vi "Build Waveform Settings.vi"(8 "error in":errorcluster, 11 "Node Ptr":T1 format="%.0x") -> (0 "error out":errorcluster, 2 "Waveform Settings Table":string[][](array[string]), 3 "Node Ptr out":T1=18446744073709551615 format="%.0x")   [LabVIEW 2026, in "SystemMonitor System Explorer.lvlib"]
uses:
  SystemMonitor System Explorer.lvlib
  <vilib>/NI VeriStand/Custom Device API/Custom Device API.lvlib
  <vilib>/NI VeriStand/Custom Device API/Custom Device Item Ref.ctl
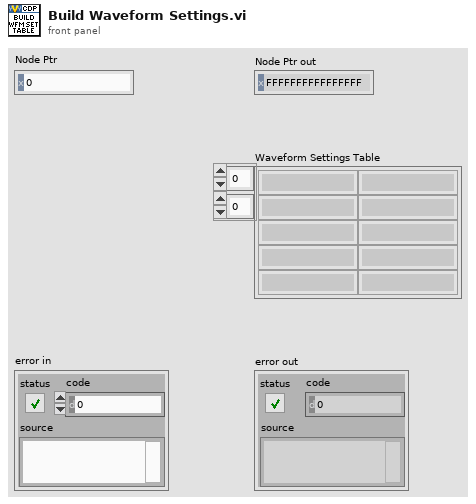
[diagram p1: front panel]
types:
  T1 = typedef "Custom Device API.lvlib/Custom Device Item Ref.ctl" = u64
  T2 = typedef "Custom Device API.lvlib/Custom Device Waveform.ctl" = cluster{"Data Type":T3, "Units":string}
  T3 = typedef "Custom Device API.lvlib/Custom Device Waveform DataType.ctl" = enum16{"Double", "Complex Double"}
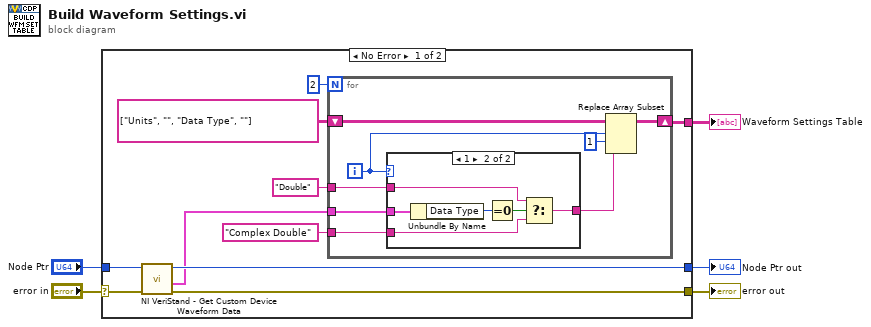
[diagram p0: block diagram]
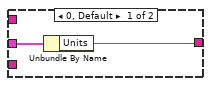
[diagram p2: hidden frame]
diagram:
  n1 = case shown="No Error" "error in" {
    selector: "error in" -> [w10 w33]
    tunnel: [w11 _] -> w5
    tunnel: [w9 w33] -> w3
    tunnel: "Node Ptr" -> [w8 w32]
    tunnel: [w7 w32] -> w1
    frame No Error {
      n2 = call <vilib>:"NI VeriStand - Get Custom Device Waveform Data.vi"("error in (no error)"=w10, "Waveform Ref in"=w8) -> ("error out"=w9:errorcluster, "Waveform"=w6:T2, "Waveform Ref out"=w7:T1)  [unwired: 4 in, 3 out]
      n3 = for {
        N: 2 -> [_]
        tunnel: w6 -> [w23]
        shift-right: [w21] -> w11
        shift-left: string[][] [["Units", ""], ["Data Type", ""]] -> [w22]
        tunnel: "Double" -> [w20]
        tunnel: "Complex Double" -> [w19]
        i -> [w17]
        n4 = case shown="1" w17 {
          tunnel: w23 -> [w25 w31]
          tunnel: w20 -> [_ w28]
          tunnel: w19 -> [_ w27]
          tunnel: [w24 w26] -> w18
          frame 0, Default {
            n5 = Unbundle By Name(w25) -> ("Units"=w24:string)
          }
          frame 1 {
            n6 = Unbundle By Name(w31) -> ("Data Type"=w30:T3)
            n7 = Equal To 0?(x=w30) -> (x = 0?=w29:bool)
            n8 = Select(t=w28, s=w29, f=w27) -> (s? t:f=w26:string)
          }
        }
        n9 = Replace Array Subset(array=w22, new element=w18, index (row)=w17, index (col)=1 ("disabled index (col)")) -> (w21:string[][])
      }
    }
    frame Error {
    }
  }
  "Waveform Settings Table" <- w5
  "error out" <- w3
  "Node Ptr out" <- w1
